vi "19.2.3-Data Matrix Code.vi"() -> ()   [LabVIEW 2017]
doc: "This example illustrates how to use the Read Data Matrix Barcode VI. There are several types of DataMatrix barcodes that are supported including ECC 000-140, ECC 200 as well as various cell shapes and barcode shapes."
uses:
  <vilib>/vision/Instrument.llb/Data Matrix Search Options.ctl
  <vilib>/vision/Instrument.llb/Demodulation Mode.ctl
  <vilib>/vision/Instrument.llb/Cell Sample Size.ctl
  <vilib>/vision/Instrument.llb/Cell Filter Mode.ctl
  <vilib>/vision/Instrument.llb/Data Matrix Size Options.ctl
  <vilib>/vision/Instrument.llb/Data Matrix Description Options.ctl
  <vilib>/vision/Instrument.llb/ECC Type.ctl
  <vilib>/vision/Instrument.llb/Data Matrix Polarity.ctl
  <vilib>/vision/Instrument.llb/Cell Fill Percentage.ctl
  <vilib>/vision/Instrument.llb/Data Matrix Mirror.ctl
  <vilib>/vision/NI_Vision_Development_Module.lvlib
panel:
  out "Read Time (ms)":dbl format="%.2f"
  out "Data":string
  out "Image":T1(plugin-control)
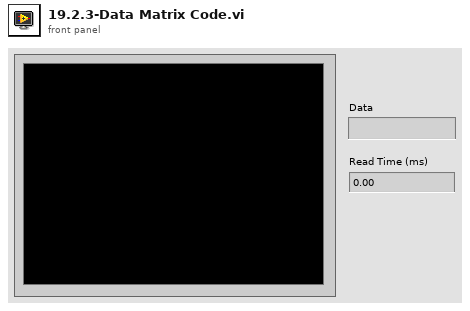
[diagram p1: front panel]
types:
  T1 = typedef "IMAQ Image.ctl" = refnum<image>
  T2 = typedef "Image Type" = u32
  T3 = typedef "Data Matrix Description Options.ctl" = cluster{"Aspect Ratio":sgl, "Rows":u32, "Columns":u32, "Rectangle":bool, "ECC":T4, "Barcode Polarity":T5, "Cell Fill Percentage":T6, "Minimum Border Integrity %":sgl, "Mirror Mode":T7}
  T4 = typedef "ECC Type.ctl" = i32
  T5 = typedef "Data Matrix Polarity.ctl" = i32
  T6 = typedef "Cell Fill Percentage.ctl" = i32
  T7 = typedef "Data Matrix Mirror.ctl" = i32
  T8 = typedef "Data Matrix Size Options.ctl" = cluster{"Data Matrix Size":cluster{"Minimum Size":u32, "Maximum Size":u32}, "Quiet Zone Width":u32}
  T9 = typedef "Data Matrix Search Options.ctl" = cluster{"Rotation Mode":enum32{"Unlimited", "0 Degrees", "90 Degrees", "180 Degrees", "270 Degrees"}, "Skip Location?":bool, "Edge Threshold":u32, "Demodulation Mode":T10, "Cell Sample Size":T11, "Cell Filter Mode":T12, "Skew Degrees Allowed":u32, "Maximum Iterations":u32, "Initial Search Vector Width":u32}
  T10 = typedef "Demodulation Mode.ctl" = i32
  T11 = typedef "Cell Sample Size.ctl" = i32
  T12 = typedef "Cell Filter Mode.ctl" = i32
  T13 = typedef "Data Matrix Report.ctl" = cluster{"Found?":bool, "Binary?":bool, "Data":string, "Bounding Box":cluster{"x":sgl, "y":sgl}[], "Errors Corrected":u32, "Erasures Corrected":u32, "Aspect Ratio":sgl, "Rows":u32, "Columns":u32, "ECC":T4, "Barcode Polarity":T5, "Cell Fill Percentage":T6, "Border Integrity":sgl, "Mirrored?":bool, "Minimum Edge Strength":u32, "Demodulation Mode":T10, "Cell Sample Size":T11, "Cell Filter Mode":T12, "Iterations":u32}
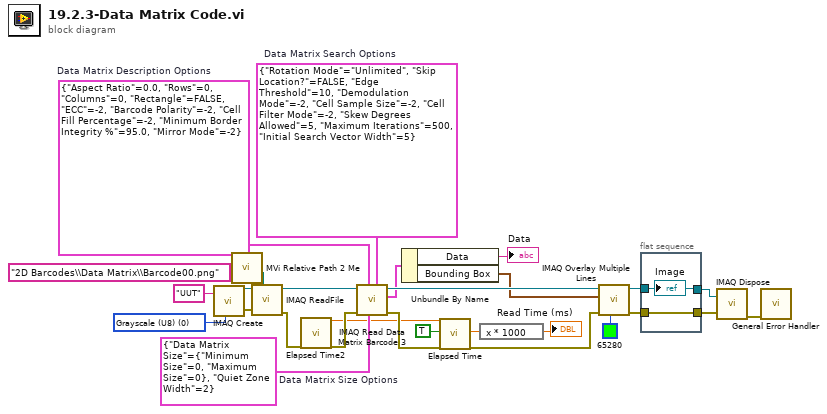
[diagram p0: block diagram]
diagram:
  w11 = T2 0 items=["Grayscale (U8)", "Grayscale (I16)", "Grayscale (SGL)", "Complex (CSG)", "RGB (U32)", "HSL (U32)", "RGB (U64)", "Grayscale (U16)"] ("Image Type")
  w19 = T3 {"Aspect Ratio"=0.0, "Rows"=0, "Columns"=0, "Rectangle"=FALSE, "ECC"=-2, "Barcode Polarity"=-2, "Cell Fill Percentage"=-2, "Minimum Border Integrity %"=95.0, "Mirror Mode"=-2}  # Data Matrix Description Options
  w18 = T8 {"Data Matrix Size"={"Minimum Size"=0, "Maximum Size"=0}, "Quiet Zone Width"=2}  # Data Matrix Size Options
  w20 = T9 {"Rotation Mode"=enum."Unlimited", "Skip Location?"=FALSE, "Edge Threshold"=10, "Demodulation Mode"=-2, "Cell Sample Size"=-2, "Cell Filter Mode"=-2, "Skew Degrees Allowed"=5, "Maximum Iterations"=500, "Initial Search Vector Width"=5}  # Data Matrix Search Options
  n1 = call "IMAQ Create"("Image Name"="UUT", "Image Type"=w11) -> ("New Image"=w9:T1, "error out"=w10:errorcluster)  [unwired: 3 in]
  n2 = call "MVi Relative Path 2 Me.vi"("Relative Path"="2D Barcodes\\Data Matrix\\Barcode00.png") -> ("Appended Dir"=w8:path)  [unwired: 5 in, 1 out]
  n3 = call "IMAQ ReadFile"("File Path"=w8, "error in (no error)"=w10, "Image"=w9) -> ("error out"=w5:errorcluster, "Image Out"=w6:T1)  [unwired: 4 in, 3 out]
  n4 = call "Elapsed Time2"("error in (no error)"=w5) -> ("Present (s)"=w14:dbl, "error out"=w21:errorcluster)  [unwired: 11 in, 6 out]
  n5 = call "IMAQ Read Data Matrix Barcode 3"("Data Matrix Search Options"=w20, "Data Matrix Size Options"=w18, "Data Matrix Description Options"=w19, "error in (no error)"=w21, "Image"=w6) -> ("error out"=w16:errorcluster, "Data Matrix Report"=w22:T13, "Image (duplicate)"=w24:T1)  [unwired: 3 in, 1 out]
  n6 = Unbundle By Name(w22) -> ("Data"=→"Data":string, "Bounding Box"=w23:cluster{"x":sgl, "y":sgl}[])
  n7 = call "Elapsed Time"("Reset"=TRUE, "error in (no error)"=w16, "Set Start Time (s)"=w14) -> ("Elapsed Time (s)"=w26:dbl, "error out"=w15:errorcluster)  [unwired: 9 in, 6 out]
  n8 = expression code="x * 1000"(w26) -> (→"Read Time (ms)":dbl)
  n9 = call "IMAQ Overlay Multiple Lines"("Color"=u32 65280, "error in (no error)"=w15, "Line End Points"=w23, "Image"=w24) -> ("error out"=w3:errorcluster, "Image Out"=w28:T1)  [unwired: 6 in]
  n10 = flat-sequence {
    tunnel: w28 -> [w30]
    tunnel: [w30] -> w1
    tunnel: w3 -> [w29]
    tunnel: [w29] -> w2
    frame #0 {
      "Image" <- w30
    }
  }
  n11 = call "IMAQ Dispose"("Image"=w1, "error in (no error)"=w2) -> ("error out"=w4:errorcluster)  [unwired: 4 in]
  n12 = call <vilib>:"General Error Handler.vi"("error in (no error)"=w4) -> ()  [unwired: 10 in, 5 out]
